vi "FPGA_target_set_stop_output.vi"(11 "connector1_data":T1) -> ()   [LabVIEW 2014]
doc: "writes the pattern data to the outputs in case the pattern output is stopped"
uses:
  FPGA_32BitPattern_data_type.ctl
  <vilib>/rvi/eio/common/nirviEmuTemplateMethod_errors.vi
  <vilib>/eio/EIONode/EIONode.xnode
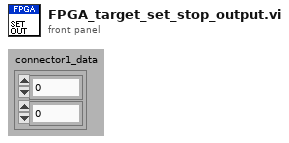
[diagram p1: front panel]
types:
  T1 = typedef "FPGA_32BitPattern_data_type.ctl" = cluster{"port0":u8, "port1":u8}
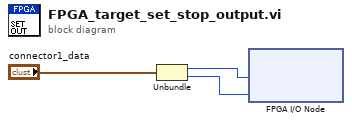
[diagram p0: block diagram]
diagram:
  n1 = Unbundle("connector1_data") -> ("port0"=w1:u8, "port1"=w2:u8)
  n2 = xnode ("FPGA I/O Node")("DO_08-15"=w1, "DO_00-07"=w2) -> ()  [unwired: 2 in, 2 out]
